vi "Edit Config.vi"(8 "error in (no error)":errorcluster, 11 "Parser in":refnum<class "Output.lvclass">) -> (0 "error out":errorcluster, 3 "Parser out":refnum<class "Output.lvclass">)   [LabVIEW 2024, in "Output.lvclass"]
doc: "Output.lvclass:Edit Config.vi\n\nThis VI is the template for the Edit Config VI for the Output class.\n\nInstrument Communication Module Version 1.0\nOctober, 2020 Original Code Consulting Davita Bird\n www.originalcode.com"
uses:
  Output.lvclass
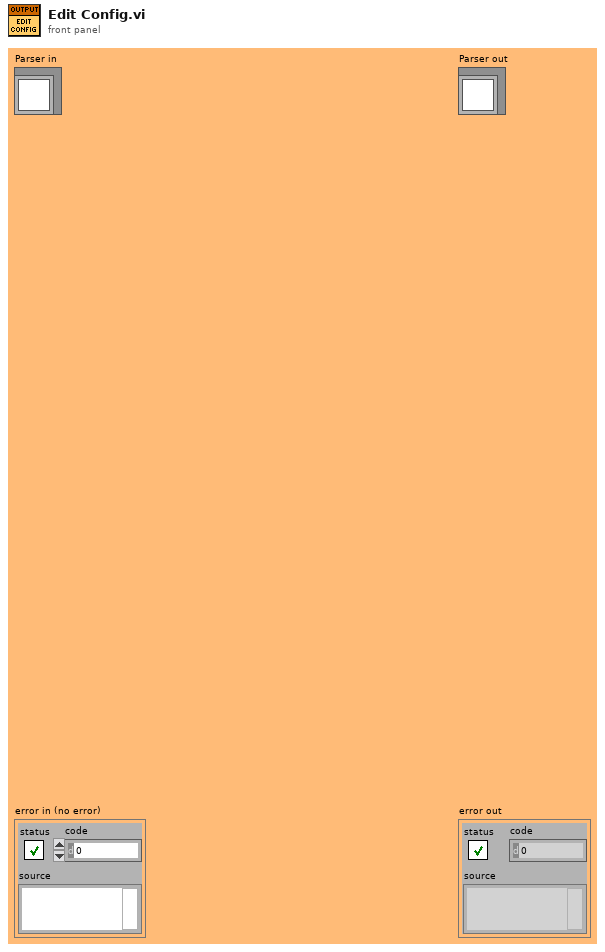
[diagram p1: front panel]
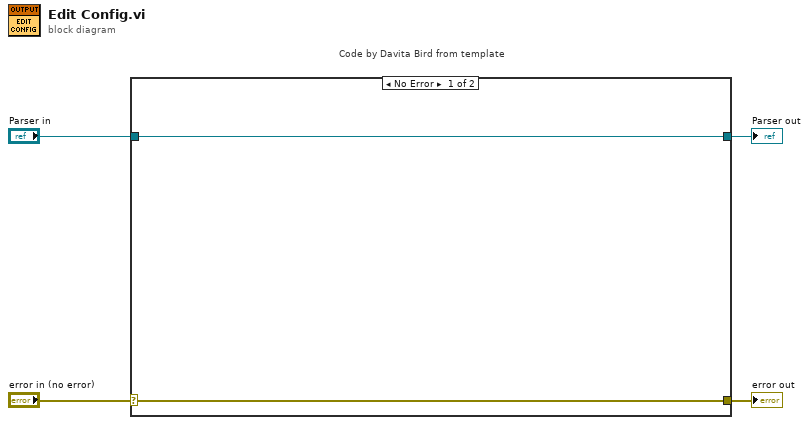
[diagram p0: block diagram]
diagram:
  n1 = case "Code by Davita Bird from template" shown="No Error" "error in (no error)" {
    selector: "error in (no error)" -> [w5 w8]
    tunnel: [w5 w8] -> w3
    tunnel: [w6 w7] -> w1
    tunnel: "Parser in" -> [w6 w7]
    frame No Error {
    }
    frame Error {
    }
  }
  "error out" <- w3
  "Parser out" <- w1
